vi "get string length in pixels.vi"(11 "notes":string) -> (3 "Numeric":i16)   [LabVIEW 2016, in "FPGA Resource Manager.lvlib"]
uses:
  FPGA Resource Manager.lvlib
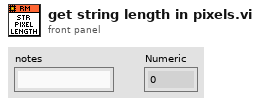
[diagram p1: front panel]
types:
  T1 = cluster{"left":i16, "top":i16, "right":i16, "bottom":i16}
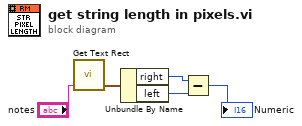
[diagram p0: block diagram]
diagram:
  n1 = call <vilib>:"Get Text Rect.vi"("text"="notes") -> ("rect"=w2:T1)  [unwired: 8 in]
  n2 = Unbundle By Name(w2) -> ("right"=w4:i16, "left"=w3:i16)
  n3 = Subtract(x=w4, y=w3) -> (x-y=→"Numeric":i16)
